vi "Msg To.vi"(9 "Insert (T) or Remove (F)":bool, 10 "Queue Nested":map{string, refnum<data-value>}(c390)) -> (3 "Update Queue Nested Msg out":refnum<class "Update Queue Nested Msg.lvclass">)   [LabVIEW 2021, in "jettl.lvlib" / "Update Queue Nested.lvlib" / "Update Queue Nested Msg.lvclass"]
uses:
  Update Queue Nested Msg.lvclass
  Msg/Msg.lvclass
  Update Queue Nested Msg.lvclass/Update Queue Nested Msg.ctl
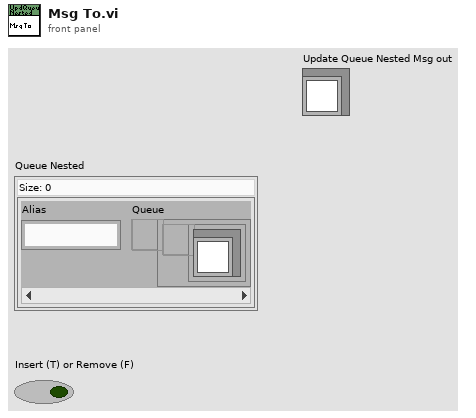
[diagram p1: front panel]
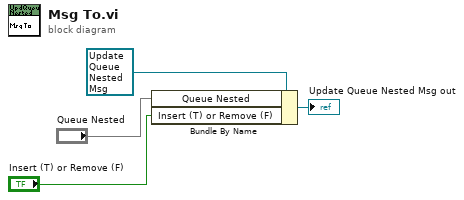
[diagram p0: block diagram]
diagram:
  n1 = Bundle By Name(cluster=refnum<class "Update Queue Nested Msg.lvclass"> refnum ("Update Queue Nested Msg out"), "Queue Nested"="Queue Nested", "Insert (T) or Remove (F)"="Insert (T) or Remove (F)") -> (→"Update Queue Nested Msg out":refnum<class "Update Queue Nested Msg.lvclass">)
